vi "VariableCheck.vi"(8 "error in (no error)":errorcluster, 9 "OriginalName":string, 10 "Variable":refnum<class "Variable.lvclass">, 11 "VariableManagerRef in":refnum<vi>) -> (0 "error out":errorcluster, 1 "RejectMessage":string, 2 "Pass":bool=TRUE, 3 "VariableManagerRef out":refnum<vi>)   [LabVIEW 2012, in "VariableManagerAPI.lvlib"]
doc: "Check the given variable definition before adding to database.\n\nReturn true if the given variable passes all tests.\nReturn false if the given variable fails some tests.\nRejectMessage can be used to identify the failed tests.\n\nThe following will make a variable definition fails the test:\n1. The difinition has an empty name\n2. The variable is set to be sequenced but the sequence function is not specified.\n3. The name is already used by another sequence index.\n4. The name is already used by another variable. Providing OriginalName will bypass the check against the given OriginalName\n5. The name begins with number.\n6. The name is t or f (reserved variable name)"
uses:
  VariableManagerAPI.lvlib
  VariableManager/VariableManager.lvclass
  Variable/Variable.lvclass
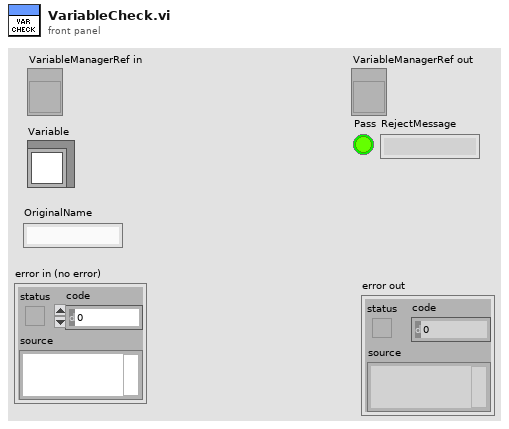
[diagram p1: front panel]
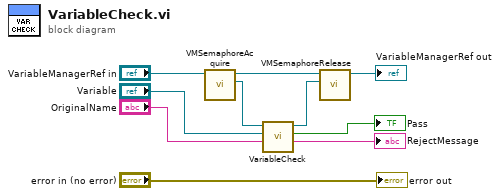
[diagram p0: block diagram]
diagram:
  n1 = call "VMSemaphoreAcquire.vi"("VariableManagerRef in"="VariableManagerRef in") -> ("VariableManager"=w5:refnum<class "VariableManager.lvclass">, "VariableManagerRef out"=w9:refnum<vi>)  [unwired: 7 in, 2 out]
  n2 = call-dynamic "VariableCheck.vi"("OriginalName"="OriginalName", "VariableIn"="Variable", "VariableManager in"=w5) -> ("RejectMessage"=→"RejectMessage":string, "Pass"=→"Pass":bool, "VariableManager out"=w6:refnum<class "VariableManager.lvclass">)  [unwired: 5 in, 1 out]
  n3 = call "VMSemaphoreRelease.vi"("VariableManager"=w6, "VariableManagerRef in"=w9) -> ("VariableManagerRef out"=→"VariableManagerRef out":refnum<vi>)  [unwired: 8 in, 1 out]
  "error out" <- "error in (no error)"
